vi "LVClass_Image ctor from copy.vi"(0 "Image in":refnum<class "Image.lvclass">, 7 "Image to copy":refnum<class "Image.lvclass">, 11 "error in (no error)":errorcluster) -> (4 "Image out":refnum<class "Image.lvclass">, 15 "error out":errorcluster)   [LabVIEW 2020, in "Image.lvclass"]
doc: "Single channel Image constructor from dimensions and bit depth.\n\n--------------------------------------------------------------------------------\n\n<B>ImageIn </B> : Constant Pointer to Image object.\n<B>ImageOut </B> : Constant Pointer to Image object.\n<B>size </B> : 2D image size.\n<B>bit_depth </B> : Image bits depth.\n<B>ErrorIn </B> : Error\n<B>ErrorOut </B> : Error\n\n--------------------------------------------------------------------------------"
uses:
  Image.lvclass
  Controls/Handle creation.ctl
  Image.lvclass/Image.ctl
  LVClass_Image read Image Compat ptr.vi
  LVClass_Image Read Image.vi
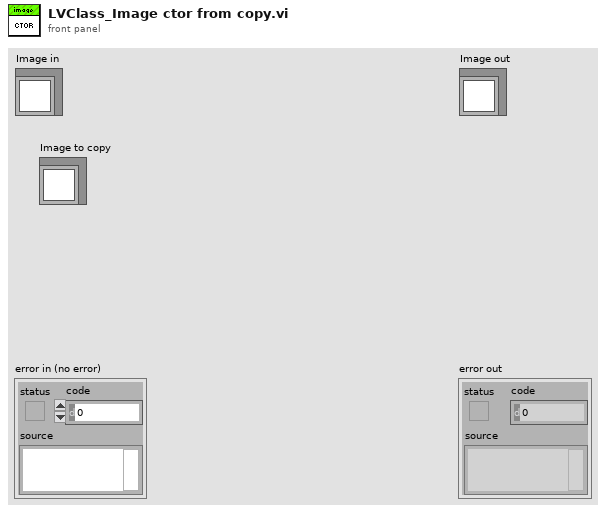
[diagram p1: front panel]
types:
  T1 = typedef "Handle creation.ctl" = enum16{"By ctor", "By write function"}
  T2 = typedef "ClassID.ctl" = i64
  T3 = typedef "Struct_Image.ctl" = cluster{"Image_Handler":T2, "Number of bits":T4, "ImageSize":T5}
  T4 = typedef "Data alignment enum.ctl" = enum16{"8", "16", "32"}
  T5 = typedef "Point2D.ctl" = cluster{"X":u32, "Y":u32}
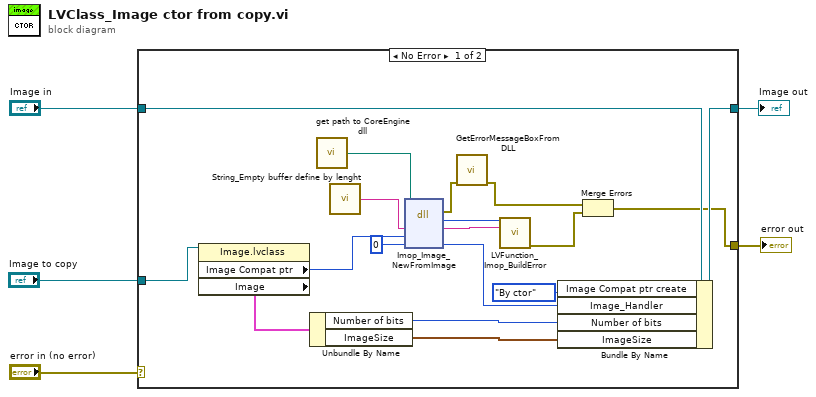
[diagram p0: block diagram]
diagram:
  n1 = case shown="No Error" "error in (no error)" {
    selector: "error in (no error)" -> [_ w25]
    tunnel: [w11 w25] -> w4
    tunnel: [w19 w24] -> w2
    tunnel: "Image in" -> [w20 w24]
    tunnel: "Image to copy" -> [w10 _]
    frame No Error {
      n2 = property class="Image.lvclass"(reference=w10) -> ("Image Compat ptr"=w9:T2, "Image"=w8:T3)  [unwired: 1 in, 2 out]
      n3 = Unbundle By Name(w8) -> ("Number of bits"=w7:T4, "ImageSize"=w6:T5)
      n4 = call "get path to CoreEngine dll.vi"() -> ("path to wavekit library"=w16:path)  [unwired: 14 in, 1 out]
      n5 = call "String_Empty buffer define by lenght.vi"() -> ("Empty buffer"=w21:string)  [unwired: 1 in]
      n6 = dll-call lib="D:/soft/HASO_v3/SVN_trunk/ImOpCoreEngine4_LV2011/DLLs/c_interface_vc100.dll" fn="Imop_Image_NewFromImage"(path in=w16, "message"=w21, "Image to copy"=w9, "NewImage"=0 ("Image compat")) -> (error out=w15:errorcluster, "return type"=w22:i32, "message"=w23:string, "NewImage"=w14:i64)  [unwired: 3 in, 1 out]
      n7 = call "GetErrorMessageBoxFromDLL.vi"("error IN"=w15) -> ("error OUT"=w13:errorcluster)  [unwired: 10 in]
      n8 = call "LVFunction_Imop_BuildError.vi"("code"=w22, "String to Prepend to source (\"\")"=w23) -> ("error out"=w12:errorcluster)  [unwired: 13 in]
      n9 = Bundle By Name(cluster=w20, "Image Compat ptr create"=Handle_creation."By ctor", "Image_Handler"=w14, "Number of bits"=w7, "ImageSize"=w6) -> (w19:refnum<class "Image.lvclass">)
      n10 = Merge Errors(w13, w12) -> (w11:errorcluster)
    }
    frame Error {
    }
  }
  "error out" <- w4
  "Image out" <- w2
